vi "reverse fft COMPLEX output.vi"(1 "samples":i32=128, 2 "fundamental frequency":dbl, 3 "fft output":cdb[](array[numeric])) -> (0 "Reversed FFT COMPLEX O/P":T1)   [LabVIEW 2009]
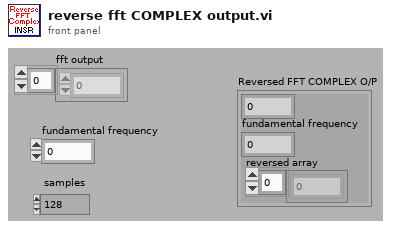
[diagram p1: front panel]
types:
  T1 = cluster{dbl, "fundamental frequency":dbl, "reversed array":cdb[]}
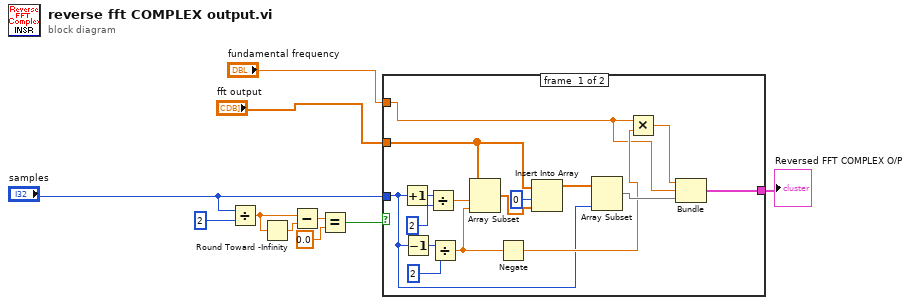
[diagram p0: block diagram]
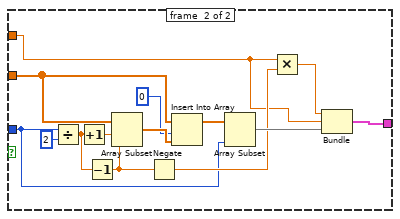
[diagram p2: hidden frame]
diagram:
  n1 = Divide(x="samples", y=2) -> (x/y=w8:dbl)
  n2 = Round Toward -Infinity(1:w8) -> (0:w9:dbl)
  n3 = Subtract(x=w8, y=w9) -> (x-y=w7:dbl)
  n4 = Equal?(x=w7, y=0.0) -> (x = y?=w5:bool)
  n5 = case shown="False" w5 {
    tunnel: "fft output" -> [w21 w37]
    tunnel: "samples" -> [w11 w27]
    tunnel: [w15 w31] -> w2
    tunnel: "fundamental frequency" -> [w12 w28]
    frame #0 {
      n6 = Increment(x=w11) -> (x+1=w26:i32)
      n7 = Decrement(x=w11) -> (x-1=w23:i32)
      n8 = Divide(x=w26, y=2) -> (x/y=w24:dbl)
      n9 = Divide(x=w23, y=2) -> (x/y=w16:dbl)
      n10 = Array Subset(array=w21, index=w24, length=w16) -> (w19:cdb[])
      n11 = Negate(x=w16) -> (-x=w14:dbl)
      n12 = Insert Into Array(array=w21, index=0, new element=w19) -> (w18:cdb[])
      n13 = Array Subset(array=w18, length=w11) -> (w17:cdb[])  [unwired: 1 in]
      n14 = Multiply(x=w12, y=w14) -> (x*y=w13:dbl)
      n15 = Bundle(w13, "fundamental frequency"=w12, w17) -> (w15:cluster{dbl, "fundamental frequency":dbl, cdb[]})  [unwired: 1 in]
    }
    frame #1 {
      n16 = Divide(x=w27, y=2) -> (x/y=w38:dbl)
      n17 = Increment(x=w38) -> (x+1=w39:dbl)
      n18 = Decrement(x=w38) -> (x-1=w32:dbl)
      n19 = Array Subset(array=w37, index=w39, length=w32) -> (w36:cdb[])
      n20 = Negate(x=w32) -> (-x=w30:dbl)
      n21 = Insert Into Array(array=w37, index=0, new element=w36) -> (w34:cdb[])
      n22 = Array Subset(array=w34, length=w27) -> (w33:cdb[])  [unwired: 1 in]
      n23 = Multiply(x=w28, y=w30) -> (x*y=w29:dbl)
      n24 = Bundle(w29, "fundamental frequency"=w28, w33) -> (w31:cluster{dbl, "fundamental frequency":dbl, cdb[]})  [unwired: 1 in]
    }
  }
  "Reversed FFT COMPLEX O/P" <- w2
